vi "goal_subst.vi"(6 "Reset":bool, 7 "Parameters":T1={"Stimulus"={"Type"=enum."Off", "Phase"=0.0, "Amplitude"=[], "Injection point"=enum."Total pose", "Closed loop"=FALSE, "Offset"=[], "Tip -> world"=FALSE, "Frequency"=0.0, "Length"=0.0}, "Goal Filter A"={"Speedup max"=0.0, "Speedup thresh"=0.0, "Speedup nonlin"=0.0, "Filters"=[]}, "Mode controls"={"Hold"=FALSE, "Cancellation"=FALSE, "Goal filter"=FALSE, "Trigger"=FALSE}, "Manipulator type"=enum."Current piezo", "Manipulator calibration"={"Tool offsets"=[[0.0, 0.0, 36200.0]], "Handle light calibration"=[], "Base pivots"=[], "Output pivots"=[], "Length center"=0.0, "Workspace height"=[], "Workspace diameter"=[0.0, 0.0, 36200.0], "Stack travel"=400.0, "Saturation pos"=375.0, "Inverse filters"=[], "Strut length"=0.0}, "Network"={"Remote Host"="", "Send Status"=FALSE, "Send Port"=0, "Recv Commands"=FALSE, "Recv Port"=0}, "Goal Filter B"={"Speedup max"=0.0, "Speedup thresh"=0.0, "Speedup nonlin"=0.0, "Filters"=[]}, "Cancellation"={"KP"={"XY"=0.0, "Rxy"=0.0, "Z"=0.0, "Rz"=0.0}, "KI"=0.0, "KD"={"XY"=0.0, "Rxy"=0.0, "Z"=0.0, "Rz"=0.0}, "Max vel"=20.0, "Max acc"=0.001, "Int error limit"=3.0, "RCM gain"=0.0, "Bypass"=FALSE, "Degraded gain"=0.0}, "Transition time"=0.0, "Estimation"={"Link"={"Measure noise"=[], "Process noise"=[], "Alt process noise"=[], "Alt turnoff cycles"=20, "Innovation limit"=[], "Residue threshold"=0.0, "Enable"=FALSE}, "Handle"={"Measure noise"=[], "Process noise"=[], "State limits"=[], "Innovation limit"=[], "Prediction Lookahead"=0.0, "Enable"=FALSE}}} {"Transition time" format="%_3f"; "Cancellation"."Degraded gain" min=0 max=1 step=0.1 format="%#_3p"; "Cancellation"."RCM gain" min=0 max=1 step=0.1 format="%#_3p"; "Cancellation"."KD"."Rz" min=-1 max=1 step=0.01 format="%#_3p"; "Cancellation"."KD"."Rxy" min=-1 max=1 step=0.01 format="%#_3p"; "Cancellation"."KD"."Z" min=-1 max=1 step=0.01 format="%#_3p"; "Cancellation"."KD"."XY" min=-1 max=1 step=0.01 format="%#_3p"; "Cancellation"."KI" min=0 max=1 step=0.01 format="%#_3p"; "Cancellation"."KP"."Rz" min=-1 max=1 step=0.01 format="%#_3p"; "Cancellation"."KP"."Rxy" min=-1 max=1 step=0.01 format="%#_3p"; "Cancellation"."KP"."Z" min=-1 max=1 step=0.01 format="%#_3p"; "Cancellation"."KP"."XY" min=-1 max=1 step=0.01 format="%#_3p"; "Cancellation"."Max acc" format="%#_3p"; "Goal Filter B"."Filters"."V limit range" format="%_3p"; "Goal Filter B"."Filters"."V limit" format="%_3p"; "Goal Filter B"."Filters"."Upper Q" format="%_3f"; "Goal Filter B"."Filters"."Upper Fc" format="%_3p"; "Goal Filter B"."Filters"."Lower Q" format="%_3f"; "Goal Filter B"."Filters"."Scale factor" format="%_3f"; "Goal Filter B"."Filters"."Lower Fc" format="%_3p"; "Goal Filter B"."Speedup nonlin" format="%_3p"; "Goal Filter B"."Speedup thresh" format="%_3p"; "Goal Filter B"."Speedup max" format="%_3p"; "Manipulator calibration"."Strut length" format="%#_4p"; "Manipulator calibration"."Saturation pos" format="%#.1f"; "Manipulator calibration"."Stack travel" format="%#.1f"; "Manipulator calibration"."Length center" format="%#_4p"; "Manipulator calibration"."Output pivots" format="%#_6f"; "Manipulator calibration"."Base pivots" format="%#_6f"; "Manipulator calibration"."Handle light calibration" format="%#.1f"; "Goal Filter A"."Filters"."V limit range" format="%_3p"; "Goal Filter A"."Filters"."V limit" format="%_3p"; "Goal Filter A"."Filters"."Upper Q" format="%_3f"; "Goal Filter A"."Filters"."Upper Fc" format="%_3p"; "Goal Filter A"."Filters"."Lower Q" format="%_3f"; "Goal Filter A"."Filters"."Scale factor" format="%_3f"; "Goal Filter A"."Filters"."Lower Fc" format="%_3p"; "Goal Filter A"."Speedup nonlin" format="%_3p"; "Goal Filter A"."Speedup thresh" format="%_3p"; "Goal Filter A"."Speedup max" format="%_3p"; "Stimulus"."Length" min=0.0 max=100.0 step=100.0 format="%#_4p"; "Stimulus"."Frequency" min=0.0 step=100.0 format="%#_4g"; "Stimulus"."Offset" format="%#_3p"; "Stimulus"."Amplitude" format="%#_3p"; "Stimulus"."Phase" min=-180.0 max=360.0 step=100.0 format="%#.2f"}, 9 "Link goal":sgl[](array[numeric])) -> (1 "Substituted goal":sgl[](array[numeric]))   [LabVIEW 2014]
uses:
  testing/Micron params.ctl
  testing/stimulus.ctl
  testing/injection_point.ctl
  filtering/goal_loop_parms.ctl
  testing/mode_conrols.ctl
  testing/manipulator_cal.ctl
  asap/labview/testing/probe_calibration.ctl
  host/network_params.ctl
  sq_control_params.ctl
  decoupled_gain.ctl
  estimation_controls.ctl
panel:
  in  "Saturation mode":bool
  # "Locals:"
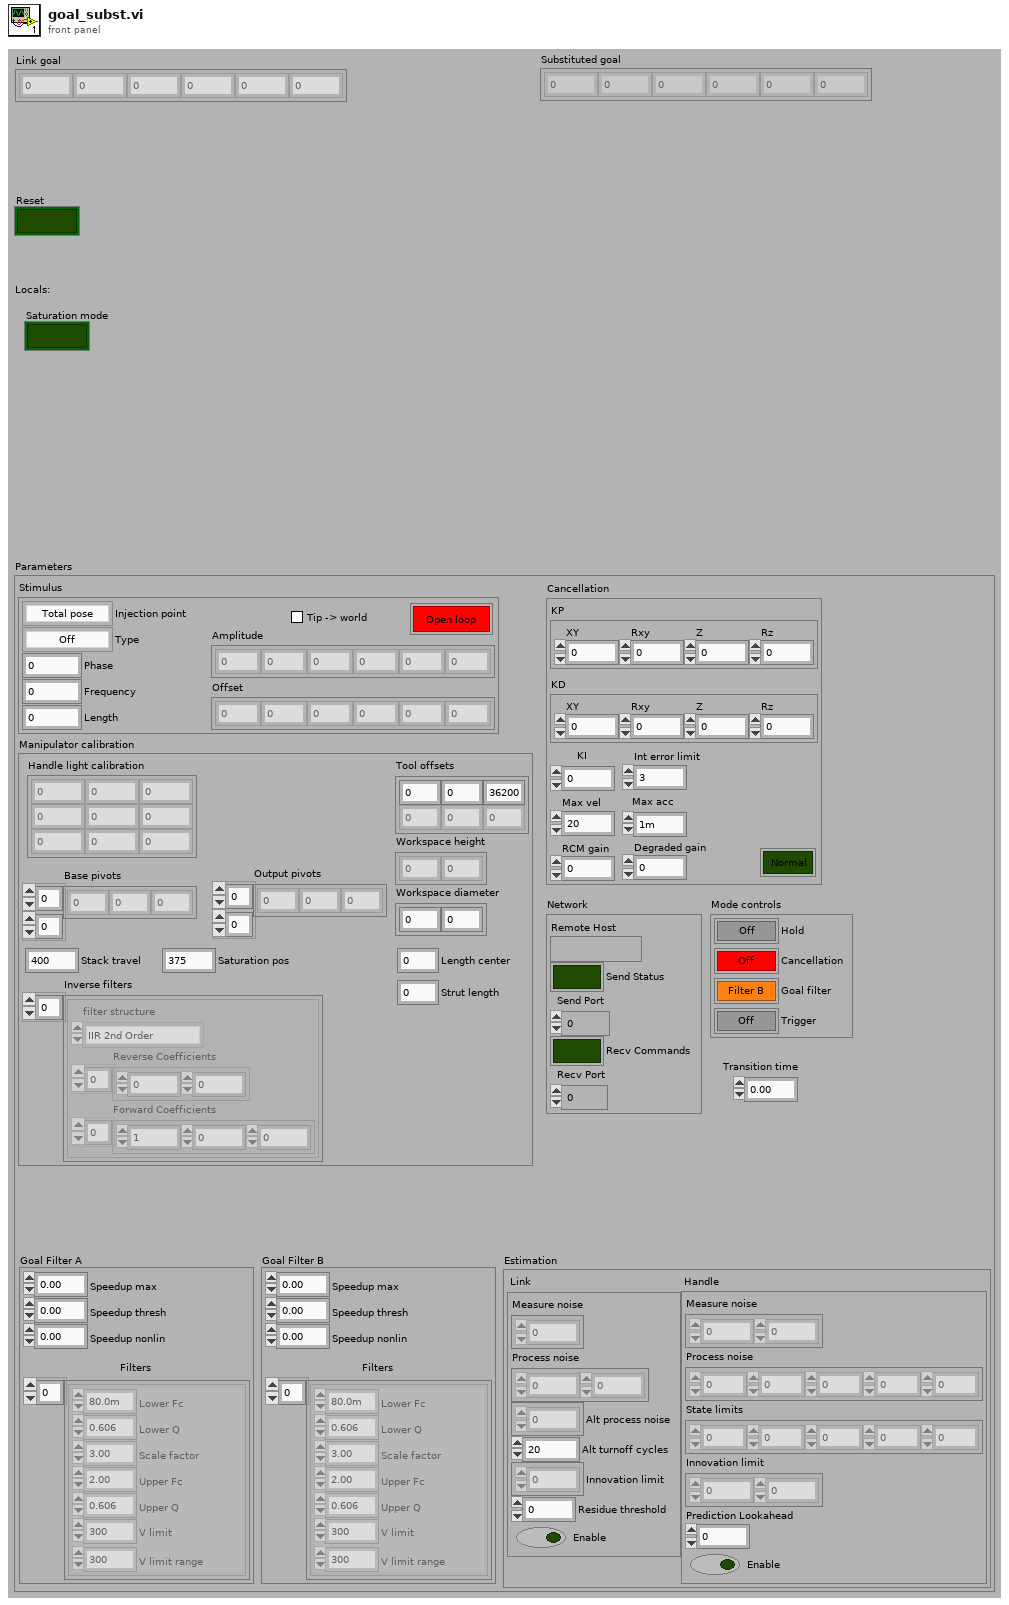
[diagram p1: front panel]
types:
  T1 = typedef "Micron params.ctl" = cluster{"Stimulus":T2, "Goal Filter A":T4, "Mode controls":T5, "Manipulator type":enum16{"Current piezo", "Voltage piezo"}, "Manipulator calibration":T6, "Network":T8, "Goal Filter B":T4, "Cancellation":T9, "Transition time":sgl, "Estimation":T11}
  T2 = typedef "stimulus.ctl" = cluster{"Type":enum16{"Off", "Step", "Sine", "Triangle", "Arbitrary"}, "Phase":dbl, "Amplitude":sgl[], "Injection point":T3, "Closed loop":bool, "Offset":sgl[], "Tip -> world":bool, "Frequency":dbl, "Length":dbl}
  T3 = typedef "injection_point.ctl" = enum16{"Total pose", "V limiter", "Goal ", "Link position", "KF link position", "Inverse kin", "Link goal", "Link error", "Controller", "Output", "Drive", "Light"}
  T4 = typedef "goal_loop_parms.ctl" = cluster{"Speedup max":sgl, "Speedup thresh":sgl, "Speedup nonlin":sgl, "Filters":cluster{"Lower Fc":sgl, "Lower Q":sgl, "Scale factor":sgl, "Upper Fc":sgl, "Upper Q":sgl, "V limit":sgl, "V limit range":sgl}[]}
  T5 = typedef "mode_conrols.ctl" = cluster{"Hold":bool, "Cancellation":bool, "Goal filter":bool, "Trigger":bool}
  T6 = typedef "manipulator_cal.ctl" = cluster{"Tool offsets":sgl[][], "Handle light calibration":T7, "Base pivots":sgl[][], "Output pivots":sgl[][], "Length center":sgl, "Workspace height":sgl[], "Workspace diameter":sgl[], "Stack travel":sgl, "Saturation pos":sgl, "Inverse filters":cluster{"filter structure":enum32{"IIR 2nd Order", "IIR 4th Order"}, "Reverse Coefficients":dbl[], "Forward Coefficients":dbl[]}[], "Strut length":sgl}
  T7 = typedef "probe_calibration.ctl" = sgl[][]
  T8 = typedef "network_params.ctl" = cluster{"Remote Host":string, "Send Status":bool, "Send Port":u16, "Recv Commands":bool, "Recv Port":u16}
  T9 = typedef "sq_control_params.ctl" = cluster{"KP":T10, "KI":sgl, "KD":T10, "Max vel":sgl, "Max acc":sgl, "Int error limit":sgl, "RCM gain":sgl, "Bypass":bool, "Degraded gain":sgl}
  T10 = typedef "decoupled_gain.ctl" = cluster{"XY":sgl, "Rxy":sgl, "Z":sgl, "Rz":sgl}
  T11 = typedef "estimation_controls.ctl" = cluster{"Link":cluster{"Measure noise":dbl[], "Process noise":dbl[], "Alt process noise":dbl[], "Alt turnoff cycles":i32, "Innovation limit":dbl[], "Residue threshold":dbl, "Enable":bool}, "Handle":cluster{"Measure noise":dbl[], "Process noise":dbl[], "State limits":dbl[], "Innovation limit":dbl[], "Prediction Lookahead":sgl, "Enable":bool}}
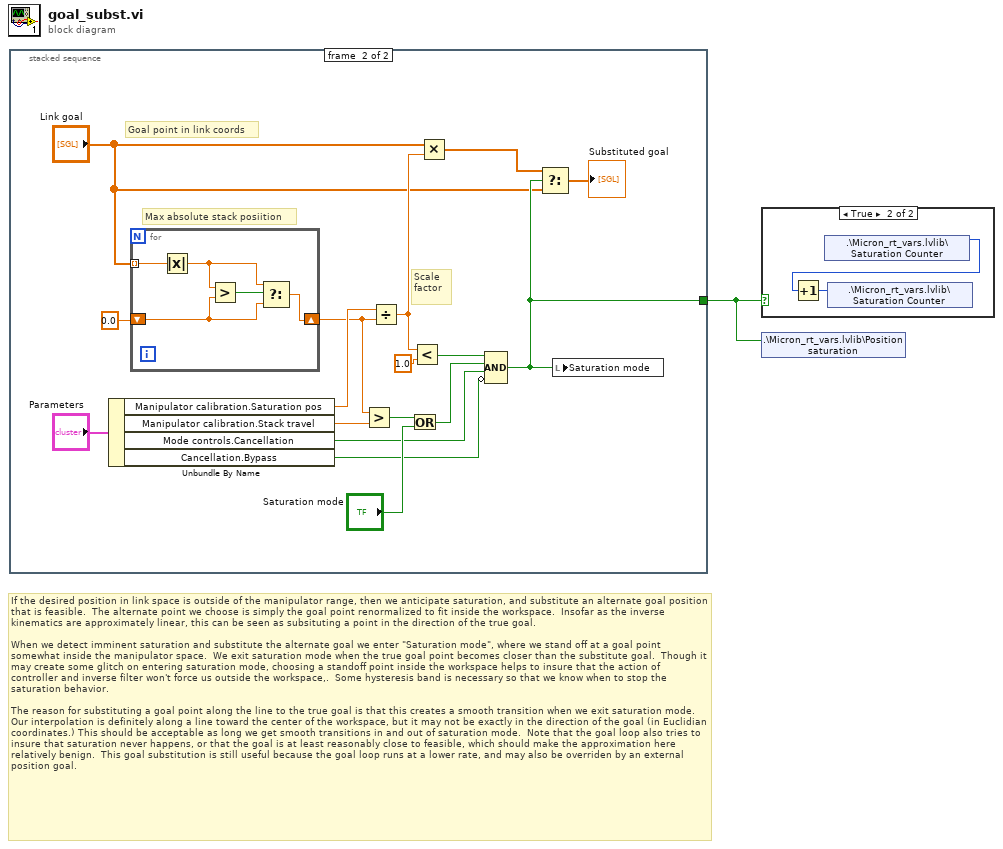
[diagram p0: block diagram]
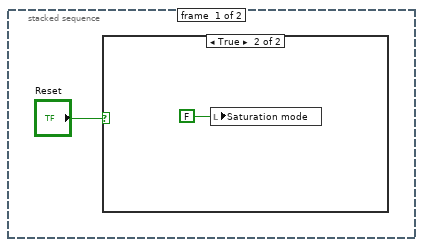
[diagram p3: hidden frame]
diagram:
  # "If the desired position in link space is outside of the manipulator range, then we anticipate saturation, and substitute an alternate goal position that is feasible.  The alternate point we choose is simply the goal point renormalized to fit inside the workspace.  Insofar as the inverse kinematics are approximately linear, this can be seen as subsituting a point in the direction of the true goal.\n\nWhen we detect imminent saturation and substitute the alternate goal we enter \"Saturation mode\", where we stand off at a goal point somewhat inside the manipulator space.  We exit saturation mode when the true goal point becomes closer than the substitute goal.  Though it may create some glitch on entering saturation mode, choosing a standoff point inside the workspace helps to insure that the action of controller and inverse filter won't force us outside the workspace,.  Some hysteresis band is necessary so that we know when to stop the saturation behavior.\n\nThe reason for substituting a goal point along the line to the true goal is that this creates a smooth transition when we exit saturation mode.   Our interpolation is definitely along a line toward the center of the workspace, but it may not be exactly in the direction of the goal (in Euclidian coordinates.) This should be acceptable as long we get smooth transitions in and out of saturation mode.  Note that the goal loop also tries to insure that saturation never happens, or that the goal is at least reasonably close to feasible, which should make the approximation here relatively benign.  This goal substitution is still useful because the goal loop runs at a lower rate, and may also be overriden by an external position goal."
  n1 = stacked-sequence {
    tunnel: [_ w10] -> w1
    frame #0 {
      n2 = case shown="True" "Reset" {
        frame False {
        }
        frame True {
          n3 = local write "Saturation mode"(FALSE ("Saturation mode")) -> ()
        }
      }
    }
    frame #1 {
      # "Scale factor"
      # "Max absolute stack posiition"
      # "Goal point in link coords"
      n4 = Unbundle By Name("Parameters") -> ("Manipulator calibration.Saturation pos"=w18:sgl, "Manipulator calibration.Stack travel"=w16:sgl, "Mode controls.Cancellation"=w9:bool, "Cancellation.Bypass"=w6:bool)
      n5 = for {
        tunnel: "Link goal" -> [w25] mode=indexing
        shift-right: [w21] -> w7
        shift-left: sgl 0.0 -> [w22]
        n6 = Absolute Value(x=w25) -> (abs(x)=w23:sgl)
        n7 = Greater?(x=w23, y=w22) -> (0:w24:bool)
        n8 = Select(t=w23, s=w24, f=w22) -> (s? t:f=w21:sgl)
      }
      n9 = Greater?(x=w7, y=w16) -> (0:w15:bool)
      n10 = Divide(x=w18, y=w7) -> (x/y=w8:sgl)
      n11 = Or(x=w15, y="Saturation mode") -> (x .or. y?=w12:bool)
      n12 = Less?(x=w8, y=sgl 1.0) -> (x < y?=w13:bool)
      n13 = Multiply(x="Link goal", y=w8) -> (x*y=w5:sgl[])
      n14 = Compound Arithmetic op=AND(w13, w12, w9, invert w6) -> (w10:bool)
      n15 = Select(t=w5, s=w10, f="Link goal") -> (s? t:f=→"Substituted goal":sgl[])
      n16 = local write "Saturation mode"(w10) -> ()
    }
  }
  n17 = case shown="True" w1 {
    frame False {
    }
    frame True {
      n18 = shared-variable ".\\Micron_rt_vars.lvlib\\Saturation Counter"() -> (w26:u32)  [unwired: 2 out]
      n19 = Increment(x=w26) -> (x+1=w27:u32)
      n20 = shared-variable ".\\Micron_rt_vars.lvlib\\Saturation Counter"(w27) -> ()  [unwired: 2 out]
    }
  }
  n21 = shared-variable ".\\Micron_rt_vars.lvlib\\Position saturation"(w1) -> ()  [unwired: 2 out]
